vi "Data Update Event.vi"(8 "error in (no error)":errorcluster, 11 "Command Handler in":refnum<class "Command Handler.lvclass">) -> (0 "error out":errorcluster)   [LabVIEW 2017, in "Command Handler.lvlib" / "Command Handler.lvclass"]
uses:
  Command Handler.lvclass
  Type Defs/Command Handler Data.ctl
  Command Handler.lvclass/Command Handler.ctl
  Command Parents/Command.lvclass
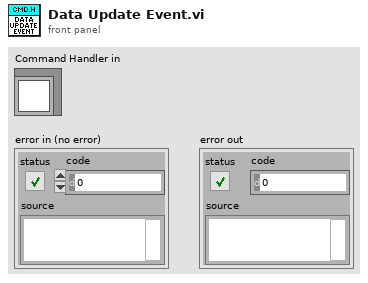
[diagram p1: front panel]
types:
  T1 = typedef "Command Handler.lvlib/Command Handler.lvclass/Command Handler Data.ctl" = cluster{"Commands Loaded":i32, "Loaded Command Names":string[], "Commands Completed":i32, "Completed Command Names":string[]}
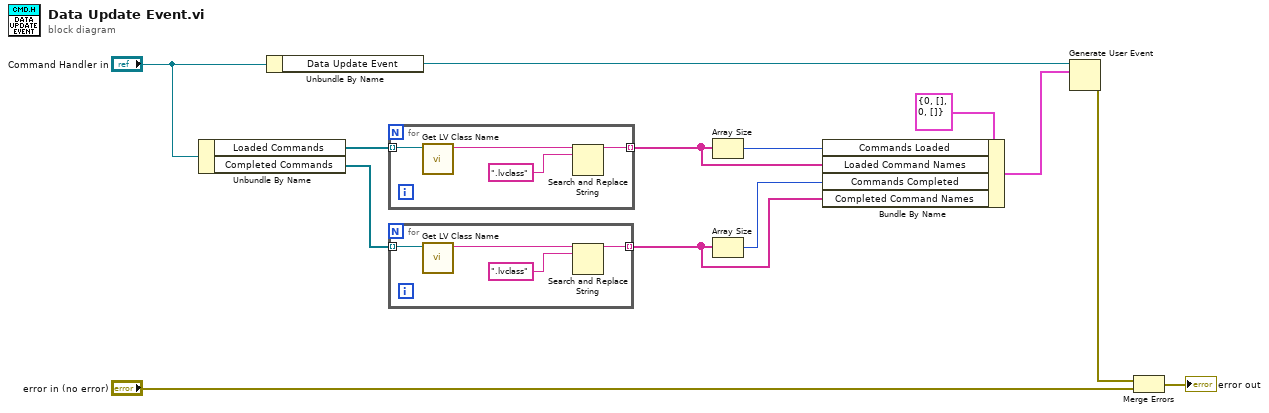
[diagram p0: block diagram]
diagram:
  n1 = Unbundle By Name("Command Handler in") -> ("Loaded Commands"=w10:refnum<class "Command.lvclass">[], "Completed Commands"=w9:refnum<class "Command.lvclass">[])
  n2 = Unbundle By Name("Command Handler in") -> ("Data Update Event"=w13:refnum<user-event>)
  n3 = for {
    tunnel: w10 -> [w17] mode=indexing
    tunnel: [w15] -> w6 mode=indexing
    n4 = call <vilib>:"Get LV Class Name.vi"("object"=w17) -> ("class name"=w16:string)  [unwired: 9 in, 1 out]
    n5 = Search and Replace String(input string=w16, search string=".lvclass") -> (result string=w15:string)  [unwired: 6 in, 3 out]
  }
  n6 = for {
    tunnel: w9 -> [w21] mode=indexing
    tunnel: [w18] -> w4 mode=indexing
    n7 = call <vilib>:"Get LV Class Name.vi"("object"=w21) -> ("class name"=w19:string)  [unwired: 9 in, 1 out]
    n8 = Search and Replace String(input string=w19, search string=".lvclass") -> (result string=w18:string)  [unwired: 6 in, 3 out]
  }
  n9 = Array Size(array=w6) -> (size(s)=w7:i32)
  n10 = Array Size(array=w4) -> (size(s)=w5:i32)
  n11 = Bundle By Name(cluster=T1 {"Commands Loaded"=0, "Loaded Command Names"=[], "Commands Completed"=0, "Completed Command Names"=[]} ("event data"), "Commands Loaded"=w7, "Loaded Command Names"=w6, "Commands Completed"=w5, "Completed Command Names"=w4) -> (w8:T1)
  n12 = Generate User Event(user event=w13, event data cluster=w8) -> (error out=w3:errorcluster)  [unwired: 2 in, 1 out]
  n13 = Merge Errors(w3, "error in (no error)") -> (→"error out":errorcluster)
